vi "Add Expected Heartbeat.vi"(6 "Timeout":u16 format="%d ms", 8 "error in":errorcluster, 9 "Period":u16 format="%d ms", 10 "Node-ID":u8, 11 "Interactor in":refnum<class "Interactor.lvclass">) -> (0 "error out":errorcluster, 3 "Interactor out":refnum<class "Interactor.lvclass">)   [LabVIEW 2020, in "Interactor.lvlib" / "Interactor.lvclass"]
uses:
  Interactor.lvclass
  Interactor.lvclass/Interactor.ctl
  CANopen Master/CANopen Master.lvclass
  Network Management UI Messages/Set Expected Heartbeat Entry Msg/Set Expected Heartbeat Entry Msg.lvclass
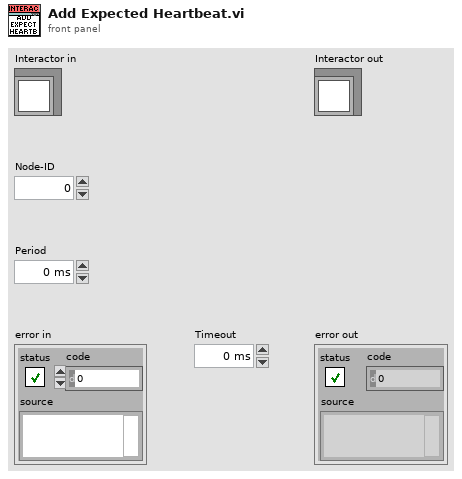
[diagram p1: front panel]
types:
  T1 = cluster{"Period":u16, "Timeout":u16, "Last Beat":timestamp}
  T2 = enum32{"Bad", "Idle", "Run top level", "Running"}
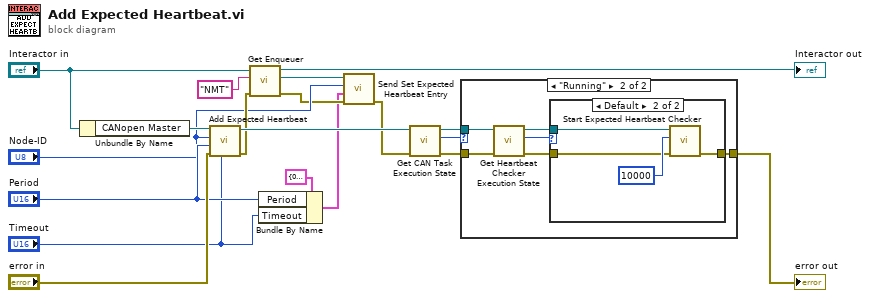
[diagram p0: block diagram]
diagram:
  n1 = Unbundle By Name("Interactor in") -> ("CANopen Master"=w19:refnum<class "CANopen Master.lvclass">)
  n2 = call "Add Expected Heartbeat.vi"("Timeout"="Timeout", "error in"="error in", "Period"="Period", "Node-ID"="Node-ID", "CANopen Master in"=w19) -> ("error out"=w10:errorcluster, "CANopen Master out"=w17:refnum<class "CANopen Master.lvclass">)  [unwired: 5 in]
  n3 = call "Get Enqueuer.vi"("error in"=w10, "Ident"="NMT", "Interactor in"="Interactor in") -> ("error out"=w3:errorcluster, "Enq"=w9:refnum<class "Message Enqueuer.lvclass">, "Interactor out"=→"Interactor out":refnum<class "Interactor.lvclass">)  [unwired: 6 in]
  n4 = Bundle By Name(cluster=T1 {"Period"=0, "Timeout"=0, "Last Beat"=timestamp(0 s since 1904-01-01)} ("Entry"), "Period"="Period", "Timeout"="Timeout") -> (w2:T1)
  n5 = call "Send Set Expected Heartbeat Entry.vi"("error in (no error)"=w3, "Entry"=w2, "Node-ID"="Node-ID", "Message Enqueuer"=w9) -> ("error out"=w1:errorcluster)  [unwired: 6 in, 1 out]
  n6 = call "Get CAN Task Execution State.vi"("error in"=w1, "CANopen Master in"=w17) -> ("error out"=w14:errorcluster, "Execution:State"=w16:T2, "CANopen Master out"=w15:refnum<class "CANopen Master.lvclass">)  [unwired: 7 in]
  n7 = case shown="\"Running\"" w16 {
    tunnel: w15 -> [_ w23]
    tunnel: w14 -> [w20 w26]
    tunnel: [w20 w25] -> w13
    frame Default {
    }
    frame "Running" {
      n8 = call "Get Heartbeat Checker Execution State.vi"("error in"=w26, "CANopen Master in"=w23) -> ("error out"=w24:errorcluster, "Execution:State"=w21:T2, "CANopen Master out"=w22:refnum<class "CANopen Master.lvclass">)  [unwired: 7 in]
      n9 = case shown="Default" w21 {
        tunnel: w22 -> [_ w31]
        tunnel: w24 -> [w27 w29]
        tunnel: [w27 w28] -> w25
        frame "Running" {
        }
        frame Default {
          n10 = call "Start Expected Heartbeat Checker.vi"("error in"=w29, "Interval"=u32 10000, "CANopen Master in"=w31) -> ("error out"=w28:errorcluster)  [unwired: 7 in, 1 out]
        }
      }
    }
  }
  "error out" <- w13
